vi "nirvififoEmulationWrite.vi"(0 "In SCTL":bool, 1 "Element":variant, 3 "Input Valid":bool, 4 "Timeout":i32, 5 "Width":i32=1024, 7 "ErrorIn":bool, 8 "Name":string="emulation", 9 "Local? (F)":bool, 10 "Is Built-In FIFO?":bool, 13 "Is Handshake?":bool, 14 "Size":i32=1024, 15 "ref in wired":bool, 16 "Type":variant, 17 "Update Size?":bool) -> (21 "Ready for Input":bool, 24 "Full":bool)   [LabVIEW 2017]
uses:
  <instcachedir>/0/nirviFifoEmulationQueueMgr_E5CAEC123FF24DC58D834DCA3CDAA9B5.lvgen/nirviFifoEmulationQueueMgr_E5CAEC123FF24DC58D834DCA3CDAA9B5_000.vi
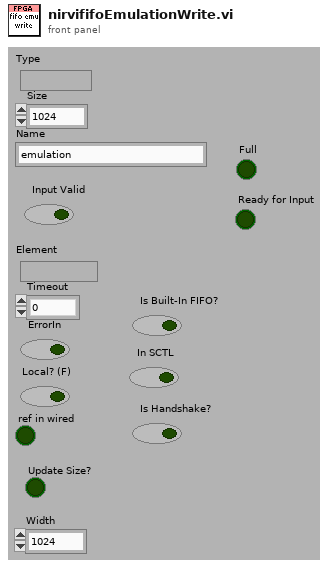
[diagram p1: front panel]
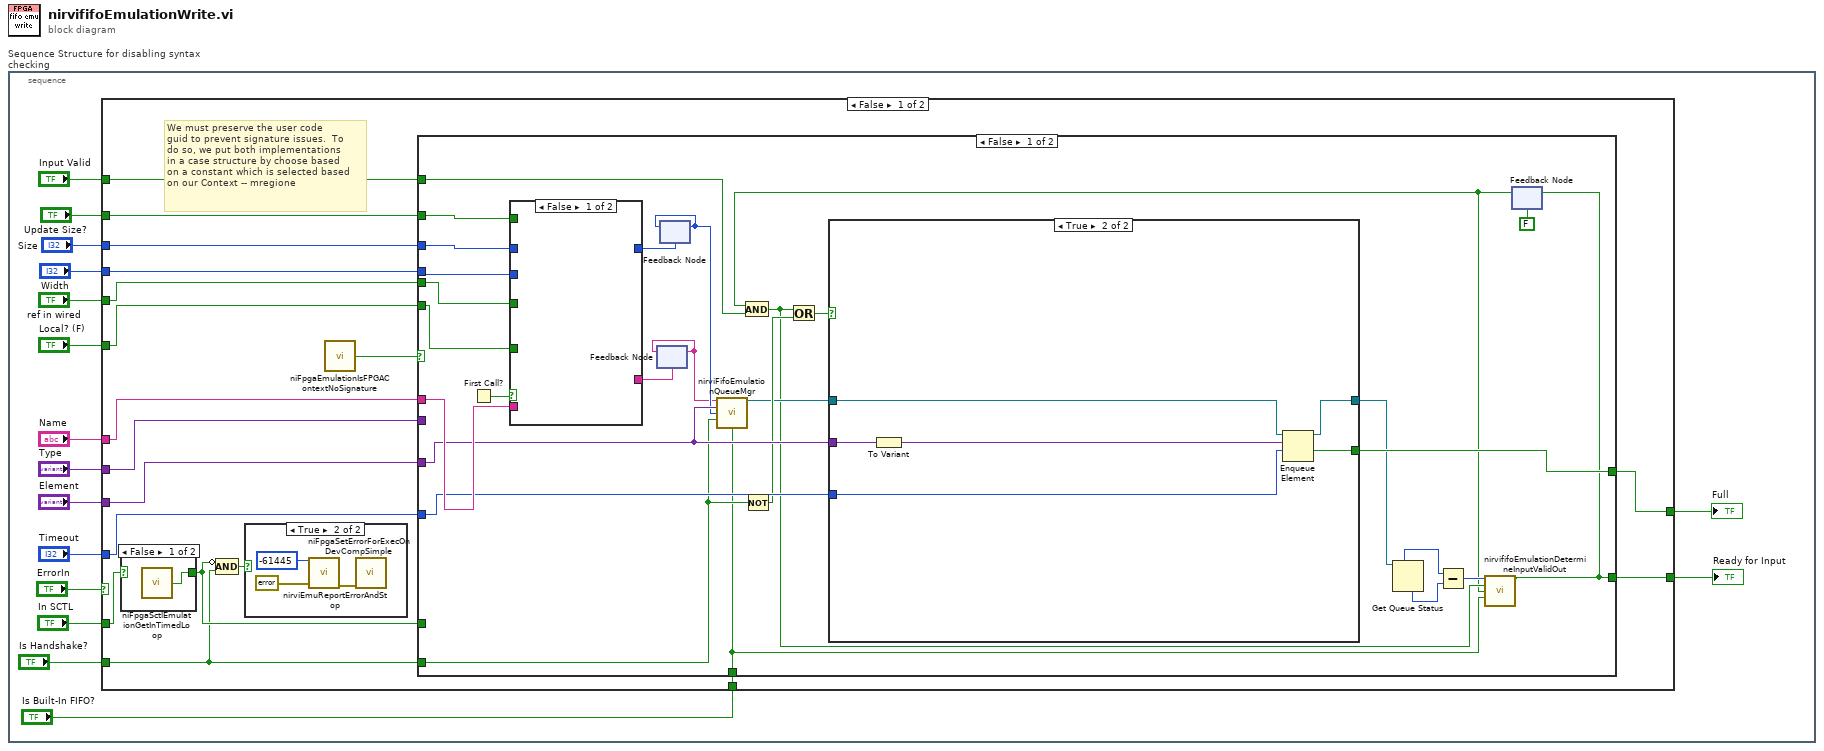
[diagram p0: block diagram]
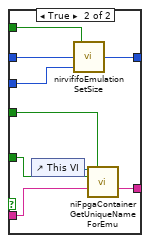
[diagram p5: hidden frame]
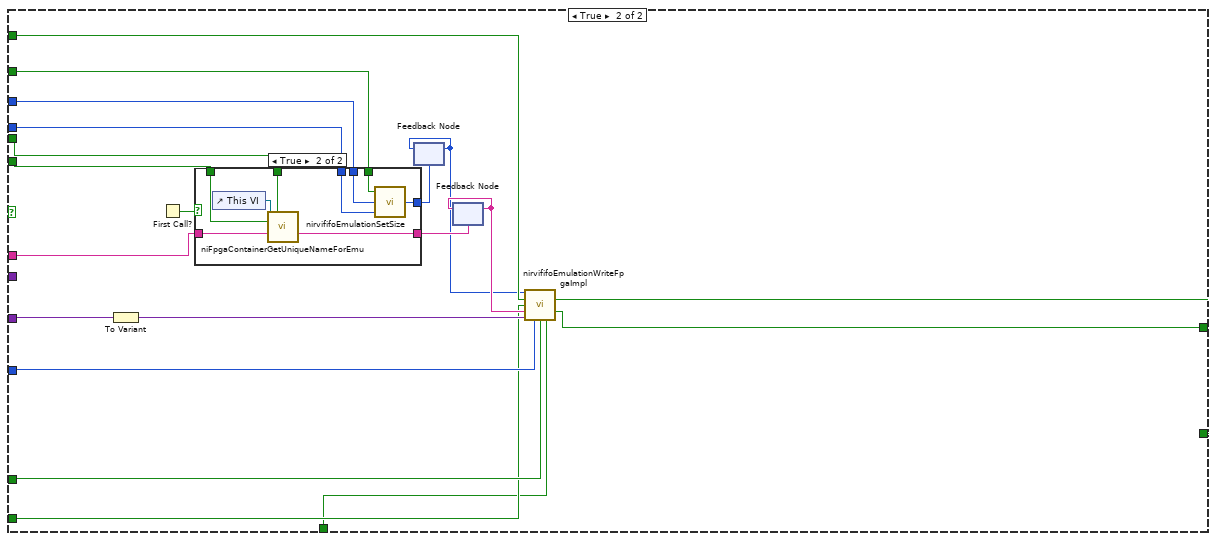
[diagram p6: hidden frame]
diagram:
  n1 = stacked-sequence "Sequence Structure for disabling syntax checking" {
    frame #0 {
      n2 = case shown="False" "ErrorIn" {
        tunnel: "Size" -> [w31 _]
        tunnel: "Name" -> [w32 _]
        tunnel: "Element" -> [w28 _]
        tunnel: "Timeout" -> [w30 _]
        tunnel: "Local? (F)" -> [w33 _]
        tunnel: "ref in wired" -> [w34 _]
        tunnel: "Update Size?" -> [w27 _]
        tunnel: "Width" -> [w26 _]
        tunnel: "In SCTL" -> [w20 _]
        tunnel: [w29 _] -> w6
        tunnel: "Type" -> [w25 _]
        tunnel: "Is Handshake?" -> [w17 _]
        tunnel: "Input Valid" -> [w23 _]
        tunnel: [w22 _] -> w2
        tunnel: "Is Built-In FIFO?" -> [w21 _]
        frame False {
          # "We must preserve the user code\nguid to prevent signature issues.  To\ndo so, we put both implementations\nin a case structure by choose based\non a constant which is selected based\non our Context -- mregione"
          n3 = case shown="False" w20 {
            selector: w20 -> [_ w36]
            tunnel: [w35 w36] -> w19
            frame False {
              n4 = call <vilib>:"niFpgaSctlEmulationGetInTimedLoop.vi"() -> ("x != 0?"=w35:bool)  [unwired: 15 in]
            }
            frame True {
            }
          }
          n5 = Compound Arithmetic op=AND(invert w19, w17) -> (w18:bool)
          n6 = case shown="True" w18 {
            frame False {
            }
            frame True {
              n7 = call <vilib>:"niFpgaSetErrorForExecOnDevCompSimple.vi"("error code"=-61445, "error in"=errorcluster {"status"=FALSE, "code"=0, "source"=""}) -> ("error out"=w37:errorcluster)  [unwired: 13 in]
              n8 = call <vilib>:"nirviEmuReportErrorAndStop.vi"("error to report"=w37) -> ()  [unwired: 1 in, 14 out]
            }
          }
          n9 = call <vilib>:"niFpgaEmulationIsFPGAContextNoSignature.vi"() -> ("Is Fpga Context?"=w24:bool)  [unwired: 15 in]
          n10 = case shown="False" w24 {
            tunnel: w34 -> [w67 w99]
            tunnel: w33 -> [w66 w98]
            tunnel: w32 -> [w65 w85]
            tunnel: w31 -> [w64 w89]
            tunnel: w19 -> [_ w95]
            tunnel: w30 -> [w63 w96]
            tunnel: [w62 w94] -> w29
            tunnel: w28 -> [w61 w97]
            tunnel: w27 -> [w60 w90]
            tunnel: w26 -> [w59 w88]
            tunnel: w25 -> [_ _]
            tunnel: w23 -> [w57 w92]
            tunnel: w17 -> [w58 w91]
            tunnel: [w43 w93] -> w22
            tunnel: w21 -> [w40 w84]
            frame False {
              n11 = First Call?() -> (First Call?: T/F=w56:bool)
              n12 = case shown="False" w56 {
                tunnel: w64 -> [_ w83]
                tunnel: w66 -> [_ w80]
                tunnel: w67 -> [_ w78]
                tunnel: w60 -> [_ w82]
                tunnel: w59 -> [_ w81]
                tunnel: [_ w76] -> w50
                tunnel: w65 -> [_ w77]
                tunnel: [_ w75] -> w52
                frame False {
                }
                frame True {
                  n13 = control-ref of="This VI"() -> (w79:refnum<vi>)
                  n14 = call <vilib>:"nirvififoEmulationSetSize.vi"("width"=w81, "Size"=w83, "Update?"=w82) -> ("Actual Size"=w75:i32)
                  n15 = call <vilib>:"niFpgaContainerGetUniqueNameForEmu.vi"("parent VI"=w79, "ref in wired"=w78, "local"=w80, "name in"=w77) -> ("name out"=w76:string)  [unwired: 11 in]
                }
              }
              n16 = feedback #1(w50) -> (w49:string)
              n17 = feedback-in #1(w49) -> ()
              n18 = feedback #2(w52) -> (w51:i32)
              n19 = feedback-in #2(w51) -> ()
              n20 = call-generic <vilib>:"nirviFifoEmulationQueueMgr.vi"("FIFO Name"=w49, "Element"=w61, "Size"=w51, "Is Handshake?"=w58, "Is Built-In FIFO?"=w40) -> ("FIFO"=w48:refnum<queue>)  [unwired: 10 in]
              n21 = Not(x=w58) -> (.not. x?=w53:bool)
              n22 = feedback #3(FALSE) -> (w41:bool)
              n23 = And(x=w41, y=w57) -> (x .and. y?=w42:bool)
              n24 = Or(x=w42, y=w53) -> (x .or. y?=w54:bool)
              n25 = case shown="True" w54 {
                tunnel: w61 -> [_ w70]
                tunnel: w63 -> [_ w74]
                tunnel: [_ w73] -> w62
                tunnel: w48 -> [w68 w72]
                tunnel: [w68 w71] -> w45
                frame False {
                }
                frame True {
                  n26 = To Variant(anything=w70) -> (Variant=w69:variant)
                  n27 = Enqueue Element(queue=w72, element=w69, timeout in ms (-1)=w74) -> (queue out=w71:refnum<queue>, timed out?=w73:bool)  [unwired: 1 in, 1 out]
                }
              }
              n28 = Get Queue Status(queue=w45) -> (max queue size=w47:i32, # elements in queue=w46:i32)  [unwired: 2 in, 6 out]
              n29 = Subtract(x=w47, y=w46) -> (x-y=w44:i32)
              n30 = call <vilib>:"nirvififoEmulationDetermineInputValidOut.vi"("Number of elements to write"=w44, "Did we write?"=w42, "Old ready for input"=w41, "Built-in?"=w40) -> ("Input Valid out"=w43:bool)  [unwired: 11 in]
              n31 = feedback-in #3(w43) -> ()
            }
            frame True {
              n32 = To Variant(anything=w97) -> (Variant=w103:variant)
              n33 = First Call?() -> (First Call?: T/F=w102:bool)
              n34 = case shown="True" w102 {
                tunnel: w99 -> [_ w111]
                tunnel: w98 -> [_ w110]
                tunnel: [_ w109] -> w101
                tunnel: w90 -> [_ w108]
                tunnel: w89 -> [_ w107]
                tunnel: w88 -> [_ w106]
                tunnel: [_ w105] -> w86
                tunnel: w85 -> [_ w104]
                frame False {
                }
                frame True {
                  n35 = control-ref of="This VI"() -> (w112:refnum<vi>)
                  n36 = call <vilib>:"niFpgaContainerGetUniqueNameForEmu.vi"("parent VI"=w112, "ref in wired"=w111, "local"=w110, "name in"=w104) -> ("name out"=w109:string)  [unwired: 11 in]
                  n37 = call <vilib>:"nirvififoEmulationSetSize.vi"("width"=w106, "Size"=w107, "Update?"=w108) -> ("Actual Size"=w105:i32)
                }
              }
              n38 = feedback #4(w86) -> (w87:i32)
              n39 = feedback-in #4(w87) -> ()
              n40 = feedback #5(w101) -> (w100:string)
              n41 = feedback-in #5(w100) -> ()
              n42 = call <vilib>:"nirvififoEmulationWriteFpgaImpl.vi"("Size"=w87, "Input Valid?"=w92, "Is Handshake?"=w91, "Name"=w100, "Init Value"=w103, "Timeout"=w96, "In Sctl?"=w95, "Is Built-In FIFO?"=w84) -> ("Ready for Input"=w93:bool, "Full?"=w94:bool)  [unwired: 6 in]
            }
          }
        }
        frame True {
        }
      }
      "Full" <- w6
      "Ready for Input" <- w2
    }
  }
